vi "Map to %.vi"(9 "In Value":dbl, 10 "low":dbl, 11 "high":dbl) -> (3 "new value":dbl)   [LabVIEW 2014]
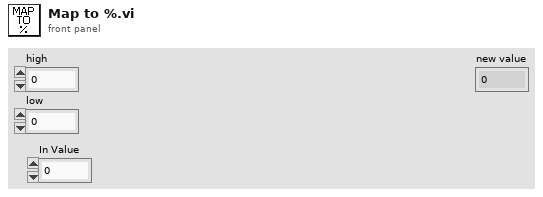
[diagram p1: front panel]
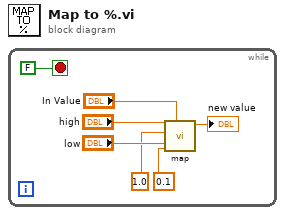
[diagram p0: block diagram]
diagram:
  n1 = while {
    stop <- FALSE stop-if-true
    n2 = call "map.vi"("value"="In Value", "new low 2"=0.1, "low"="low", "new high 2"=1.0, "high"="high") -> ("new value"=→"new value":dbl)  [unwired: 6 in]
  }
